vi "RunJS2.vi"() -> ()   [LabVIEW 2013]
uses:
  System.Windows.Forms
  E:/Dropbox/ni/lvcef/github/lvcef/dotnet/LVCef/bin/Debug/LVCef.dll
  dotnet/LVCef/bin/Debug/LVCef.dll
panel:
  in  "ToolStripContainer":refnum<k24>(container)
  out "Numeric":i32
  in  "stop":bool
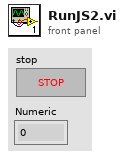
[diagram p1: front panel]
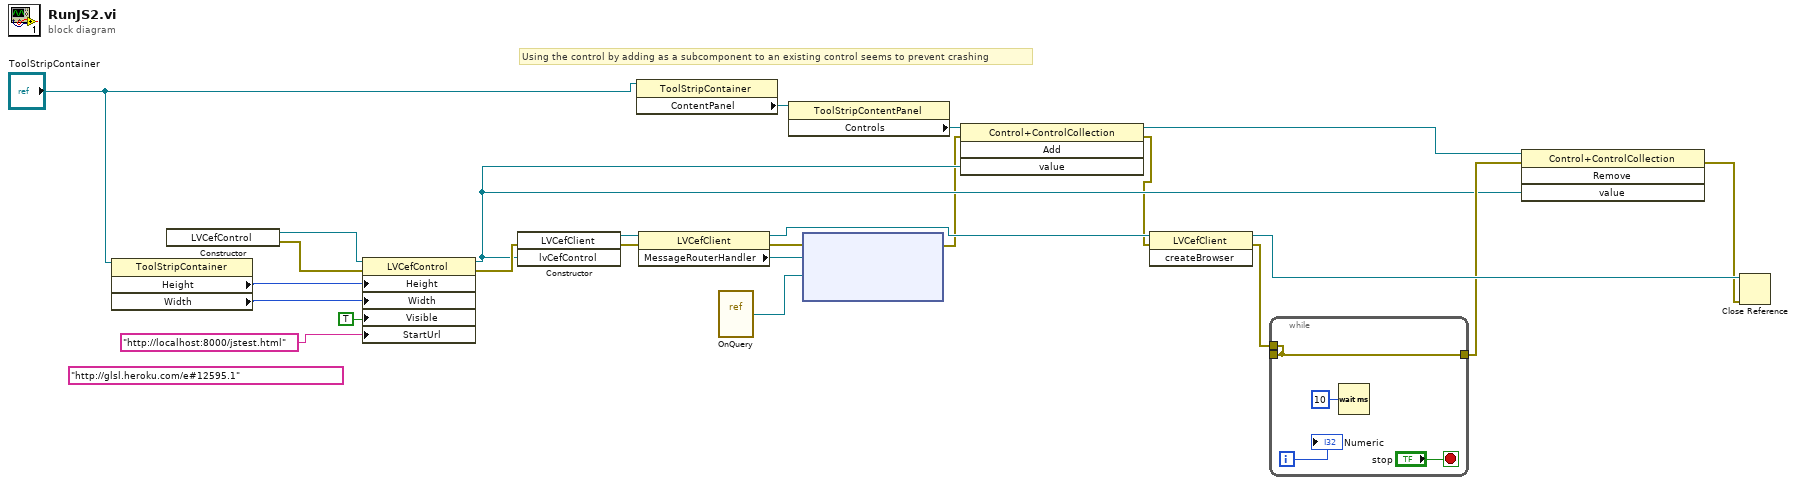
[diagram p0: block diagram]
diagram:
  (unwired) "http://glsl.heroku.com/e#12595.1" ("StartUrl")
  # "Using the control by adding as a subcomponent to an existing control seems to prevent crashing"
  n1 = property class="ToolStripContainer"(reference="ToolStripContainer") -> ("Height"=w5:i32, "Width"=w4:i32)  [unwired: 1 in, 2 out]
  n2 = constructor class="LVCefControl"() -> (reference out=w15:refnum<k24>, error out=w16:errorcluster)  [unwired: 3 in, 1 out]
  n3 = property class="LVCefControl"(reference=w15, error in=w16, "Height"=w5, "Width"=w4, "Visible"=TRUE, "StartUrl"="http://localhost:8000/jstest.html") -> (reference out=w9:refnum<k24>, error out=w23:errorcluster)
  n4 = constructor class="LVCefClient"(error in=w23, "lvCefControl"=w9) -> (reference out=w20:refnum<k24>, error out=w21:errorcluster)  [unwired: 2 in, 2 out]
  n5 = property class="ToolStripContainer"(reference="ToolStripContainer") -> ("ContentPanel"=w14:refnum<k24>)  [unwired: 1 in, 2 out]
  n6 = property class="LVCefClient"(reference=w20, error in=w21) -> (reference out=w17:refnum<k24>, error out=w19:errorcluster, "MessageRouterHandler"=w18:refnum<k24>)
  n7 = vi-ref "OnQuery.vi"() -> ("vi reference"=w1:refnum<vi>)
  n8 = property class="ToolStripContentPanel"(reference=w14) -> ("Controls"=w13:refnum<k24>)  [unwired: 1 in, 2 out]
  n9 = node(w19, w18, w1) -> (w7:errorcluster)  [unwired: 2 in, 1 out]
  n10 = invoke class="Control+ControlCollection" method="Add"(reference=w13, error in=w7, "value"=w9) -> (reference out=w10:refnum<k24>, error out=w6:errorcluster)  [unwired: 1 in, 2 out]
  n11 = invoke class="LVCefClient" method="createBrowser"(reference=w17, error in=w6) -> (reference out=w22:refnum<k24>, error out=w8:errorcluster)  [unwired: 1 in, 1 out]
  n12 = while {
    tunnel: [w25] -> _
    tunnel: [w25] -> w12
    tunnel: w8 -> [w25]
    i -> [w27]
    stop <- "stop" stop-if-true
    n13 = Wait (ms)(milliseconds to wait=u32 10) -> ()  [unwired: 1 out]
    "Numeric" <- w27
  }
  n14 = invoke class="Control+ControlCollection" method="Remove"(reference=w10, error in=w12, "value"=w9) -> (error out=w11:errorcluster)  [unwired: 1 in, 3 out]
  n15 = Close Reference(reference=w22, error in (no error)=w11) -> ()  [unwired: 1 out]
